vi "TDC_generateHbtDemo.vi"(8 "Error In":errorcluster, 9 "Noise Level":u64, 10 "Parameters":dbl[](array[numeric]), 11 "Function Type":u16(ring) items=["None", "Coherent", "Thermal", "Single", "Antibunch", "Thermal+Jitter", "Single+Jitter", "Antibunch+Jitter", "Thermal+Offset", "Single+Offset", "Antibunch+Offset", "Thermal+Jitter+Offs", "Single+Jitter+Offs", "Antibunch+Jitter+Offs"]) -> (0 "Error Out":errorcluster)   [LabVIEW 2011]
uses:
  tdcbase.dll
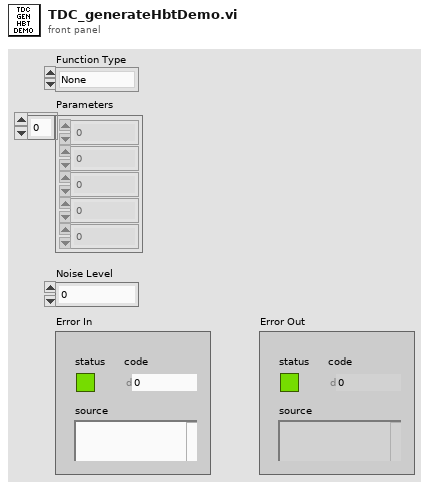
[diagram p1: front panel]
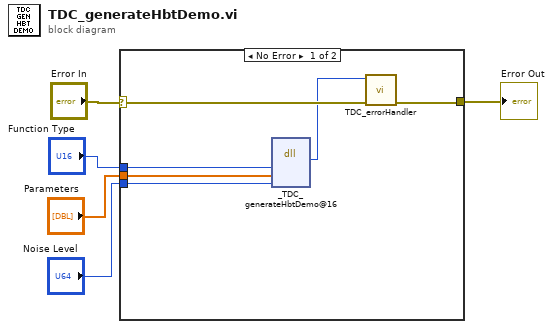
[diagram p0: block diagram]
diagram:
  n1 = case shown="No Error" "Error In" {
    selector: "Error In" -> [w11 w12]
    tunnel: [w10 w12] -> w4
    tunnel: "Function Type" -> [w8 _]
    tunnel: "Parameters" -> [w7 _]
    tunnel: "Noise Level" -> [w6 _]
    frame No Error {
      n2 = dll-call lib="X:/tdcbase.dll" fn="_TDC_generateHbtDemo@16"("fctType"=w8, "params"=w7, "noiseLv"=w6) -> ("return type"=w9:i32)  [unwired: 6 in, 2 out]
      n3 = call "TDC_errorHandler.vi"("Error In"=w11, "TDC Return Code"=w9) -> ("Error Out"=w10:errorcluster)  [unwired: 9 in]
    }
    frame Error {
    }
  }
  "Error Out" <- w4
